vi "Read.vi"(8 "error in (no error)":errorcluster, 11 "CAN_Logic in":refnum<class "CAN_Logic.lvclass">) -> (0 "error out":errorcluster, 2 "CAN Data":T1 {"payload" format="%x"; "identifier" format="%x"}, 3 "CAN_Logic out":refnum<class "CAN_Logic.lvclass">)   [LabVIEW 2021, in "CAN_Logic.lvclass"]
uses:
  CAN_Logic.lvclass
  CAN_Logic.lvclass/CAN_Logic.ctl
  <vilib>/xnet/xnet.llb/XNET Frame Type CAN.ctl
  <vilib>/xnet/xnet.llb/XNET Frame CAN.ctl
  <vilib>/xnet/xnet.llb/XNET Read (Frame CAN).vi
  Channels/ChannelRegistrar/typedef/Datatype CAN.ctl
  Channels/ChannelRegistrar/ChannelRegistrar.lvlib
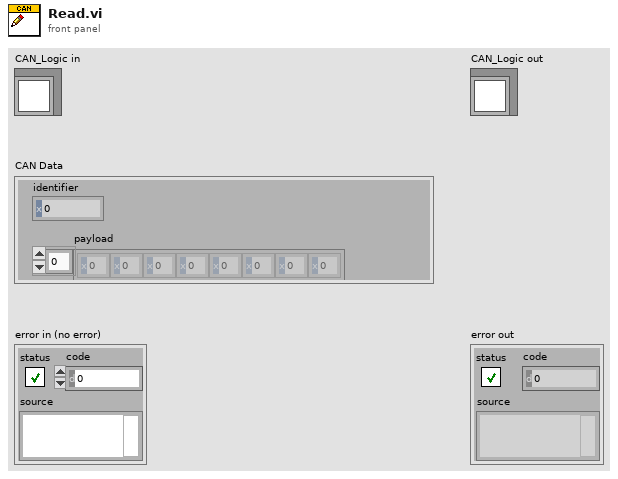
[diagram p1: front panel]
types:
  T1 = typedef "ChannelRegistrar.lvlib/Datatype CAN.ctl" = cluster{"payload":u8[], "identifier":u32}
  T2 = typedef "XNET Frame CAN.ctl" = cluster{"timestamp":timestamp, "payload":u8[], "identifier":u32, "type":T3, "extended?":bool, "echo?":bool}
  T3 = typedef "XNET Frame Type CAN.ctl" = u8
  T4 = typedef "CAN_Logic.lvclass/ISO FD Frame Type.ctl" = enum16{"Not Specified", "CAN 2.0", "FD", "FD+BRS"}
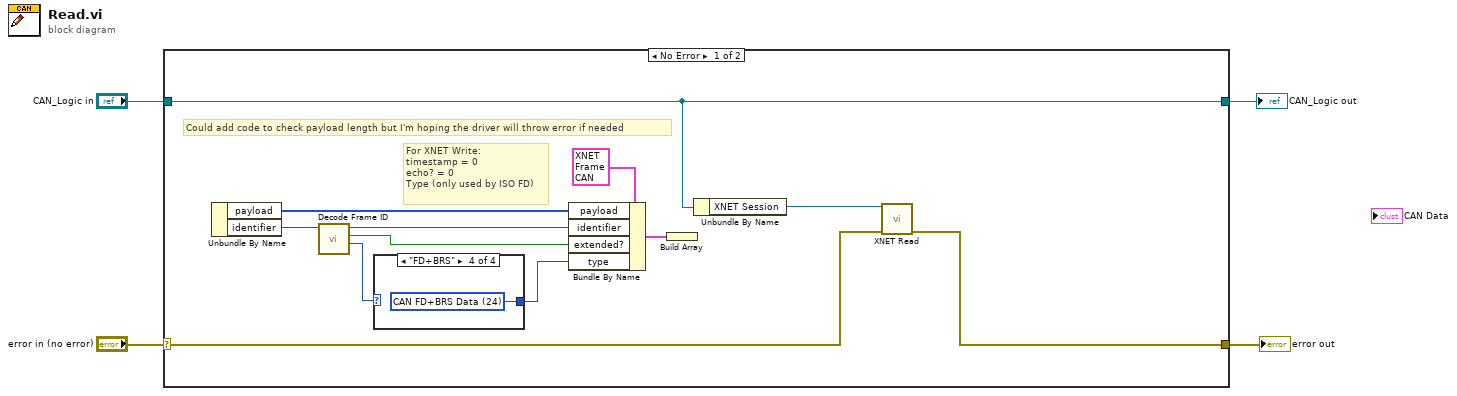
[diagram p0: block diagram]
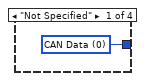
[diagram p2: hidden frame]
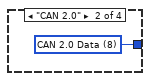
[diagram p3: hidden frame]
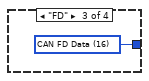
[diagram p4: hidden frame]
diagram:
  n1 = case shown="No Error" "error in (no error)" {
    selector: "error in (no error)" -> [w14 w22]
    tunnel: [w13 w22] -> w3
    tunnel: [w16 w21] -> w1
    tunnel: "CAN_Logic in" -> [w16 w21]
    frame No Error {
      # "Could add code to check payload length but I'm hoping the driver will throw error if needed"
      # "For XNET Write:\ntimestamp = 0\necho? = 0\nType (only used by ISO FD)"
      n2 = Unbundle By Name() -> ("payload"=w5:u8[], "identifier"=w10:u32)  [unwired: 1 in]
      n3 = call "Decode Frame ID.vi"("Frame ID in"=w10) -> ("ISO FD Type"=w7:T4, "Extended ID"=w8:bool, "Frame ID out"=w9:u32)  [unwired: 8 in]
      n4 = case shown="\"FD+BRS\"" w7 {
        tunnel: [w17 w18 w19 w20] -> w6
        frame "Not Specified" {
          w17 = T3 0 items=["CAN Data"=0, "CAN Remote"=1, "CAN Bus Error"=2, "CAN 2.0 Data"=8, "CAN FD Data"=16, "CAN FD+BRS Data"=24, "J1939 Data"=192, "Delay"=224, "Log Trigger"=225, "Start Trigger"=226] ("type")
        }
        frame "CAN 2.0" {
          w18 = T3 8 items=["CAN Data"=0, "CAN Remote"=1, "CAN Bus Error"=2, "CAN 2.0 Data"=8, "CAN FD Data"=16, "CAN FD+BRS Data"=24, "J1939 Data"=192, "Delay"=224, "Log Trigger"=225, "Start Trigger"=226] ("type")
        }
        frame "FD" {
          w19 = T3 16 items=["CAN Data"=0, "CAN Remote"=1, "CAN Bus Error"=2, "CAN 2.0 Data"=8, "CAN FD Data"=16, "CAN FD+BRS Data"=24, "J1939 Data"=192, "Delay"=224, "Log Trigger"=225, "Start Trigger"=226] ("type")
        }
        frame "FD+BRS" {
          w20 = T3 24 items=["CAN Data"=0, "CAN Remote"=1, "CAN Bus Error"=2, "CAN 2.0 Data"=8, "CAN FD Data"=16, "CAN FD+BRS Data"=24, "J1939 Data"=192, "Delay"=224, "Log Trigger"=225, "Start Trigger"=226] ("type")
        }
      }
      n5 = Bundle By Name(cluster=T2 {"timestamp"=timestamp(0 s since 1904-01-01), "payload"=[], "identifier"=0, "type"=0, "extended?"=FALSE, "echo?"=FALSE} ("CAN frame"), "payload"=w5, "identifier"=w9, "extended?"=w8, "type"=w6) -> (w11:T2)
      n6 = Build Array(w11) -> ()  [unwired: 1 out]
      n7 = Unbundle By Name(w16) -> ("XNET Session"=w15:refnum<k21>)
      n8 = call-poly <vilib>:"XNET Read.vi"("session in"=w15, "error in (no error)"=w14) -> ("error out"=w13:errorcluster)  [unwired: 10 in, 3 out]
    }
    frame Error {
    }
  }
  "error out" <- w3
  "CAN_Logic out" <- w1
